vi "DigitalFont.vi"() -> ()   [LabVIEW 2019, in "Digital.lvclass"]
uses:
  Digital.lvclass
  <vilib>/Analysis/coordinate.llb/2D Cartesian Coordinate Rotation (Array).vi
  <vilib>/Analysis/NI_AALPro.lvlib
panel:
  out "Array":T1(array[cluster])
  out "new picture 2":picture
  in  "Numeric":i32
  in  "TopLeft":cluster{"String":dbl, "String":dbl}[](array[cluster])=[{"String"=10.0, "String"=100.0}, {"String"=1.2246467991473533e-15, "String"=80.0}, {"String"=4.898587196589413e-15, "String"=20.0}, {"String"=10.000000000000005, "String"=0.0}, {"String"=20.000000000000004, "String"=20.0}, {"String"=20.0, "String"=80.0}, {"String"=10.0, "String"=100.0}]
  out "appended array":cluster{"String":dbl, "String":dbl}[](array[cluster])
  out "new picture":picture
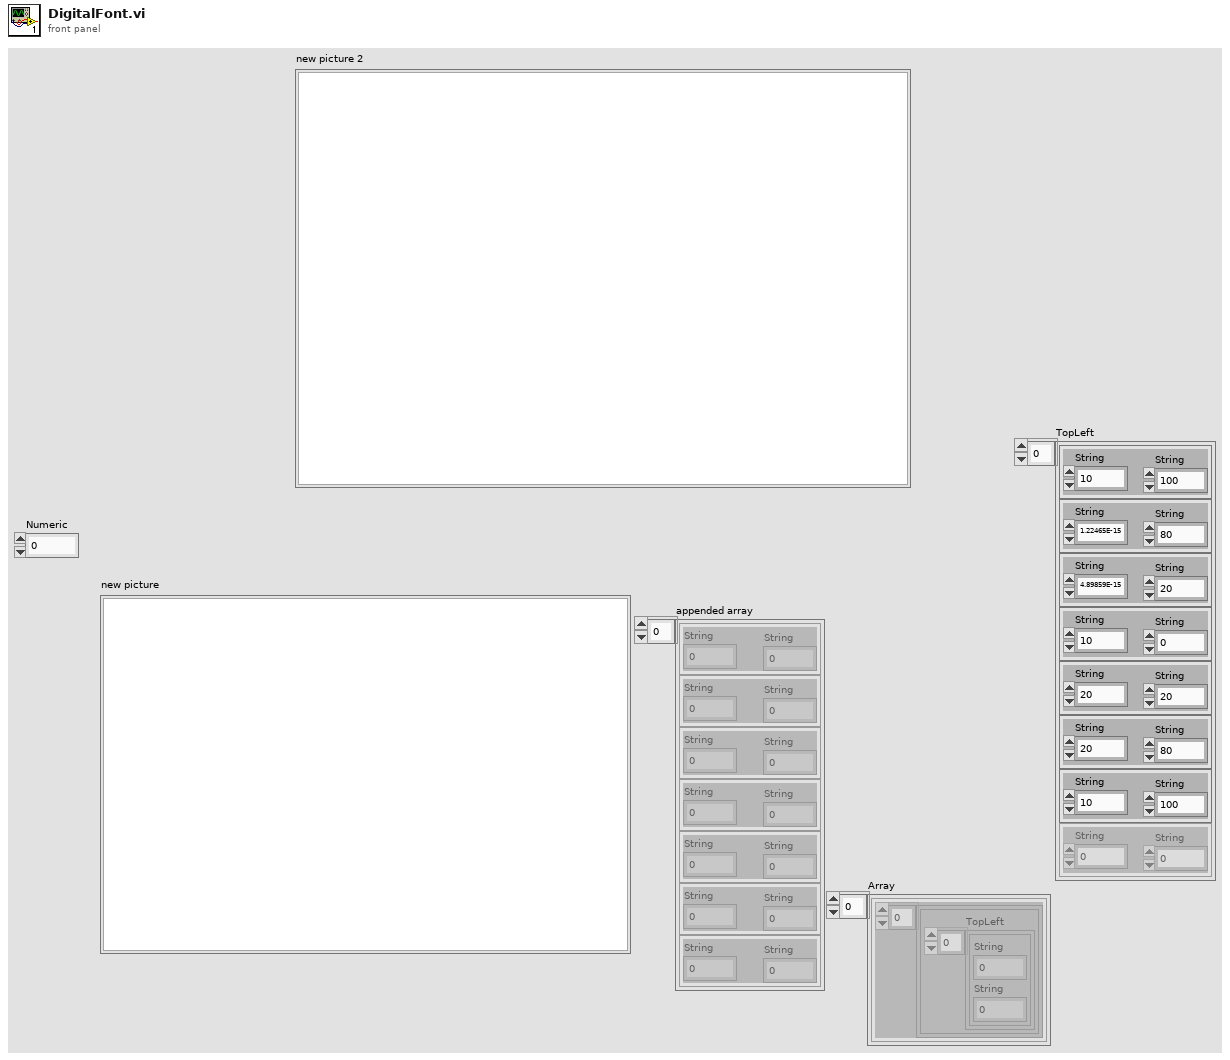
[diagram p1: front panel]
types:
  T1 = cluster{cluster{"TopLeft":cluster{"String":dbl, "String":dbl}[]}[]}[]
  T2 = cluster{"TopLeft":cluster{"String":dbl, "String":dbl}[]}[]
  T3 = cluster{"TopLeft":cluster{"String":dbl, "String":dbl}[]}
  T4 = cluster{"Width":u16, "Style":enum32{"Solid", "Dash", "Dot", "DashDot", "DashDotDot"}}
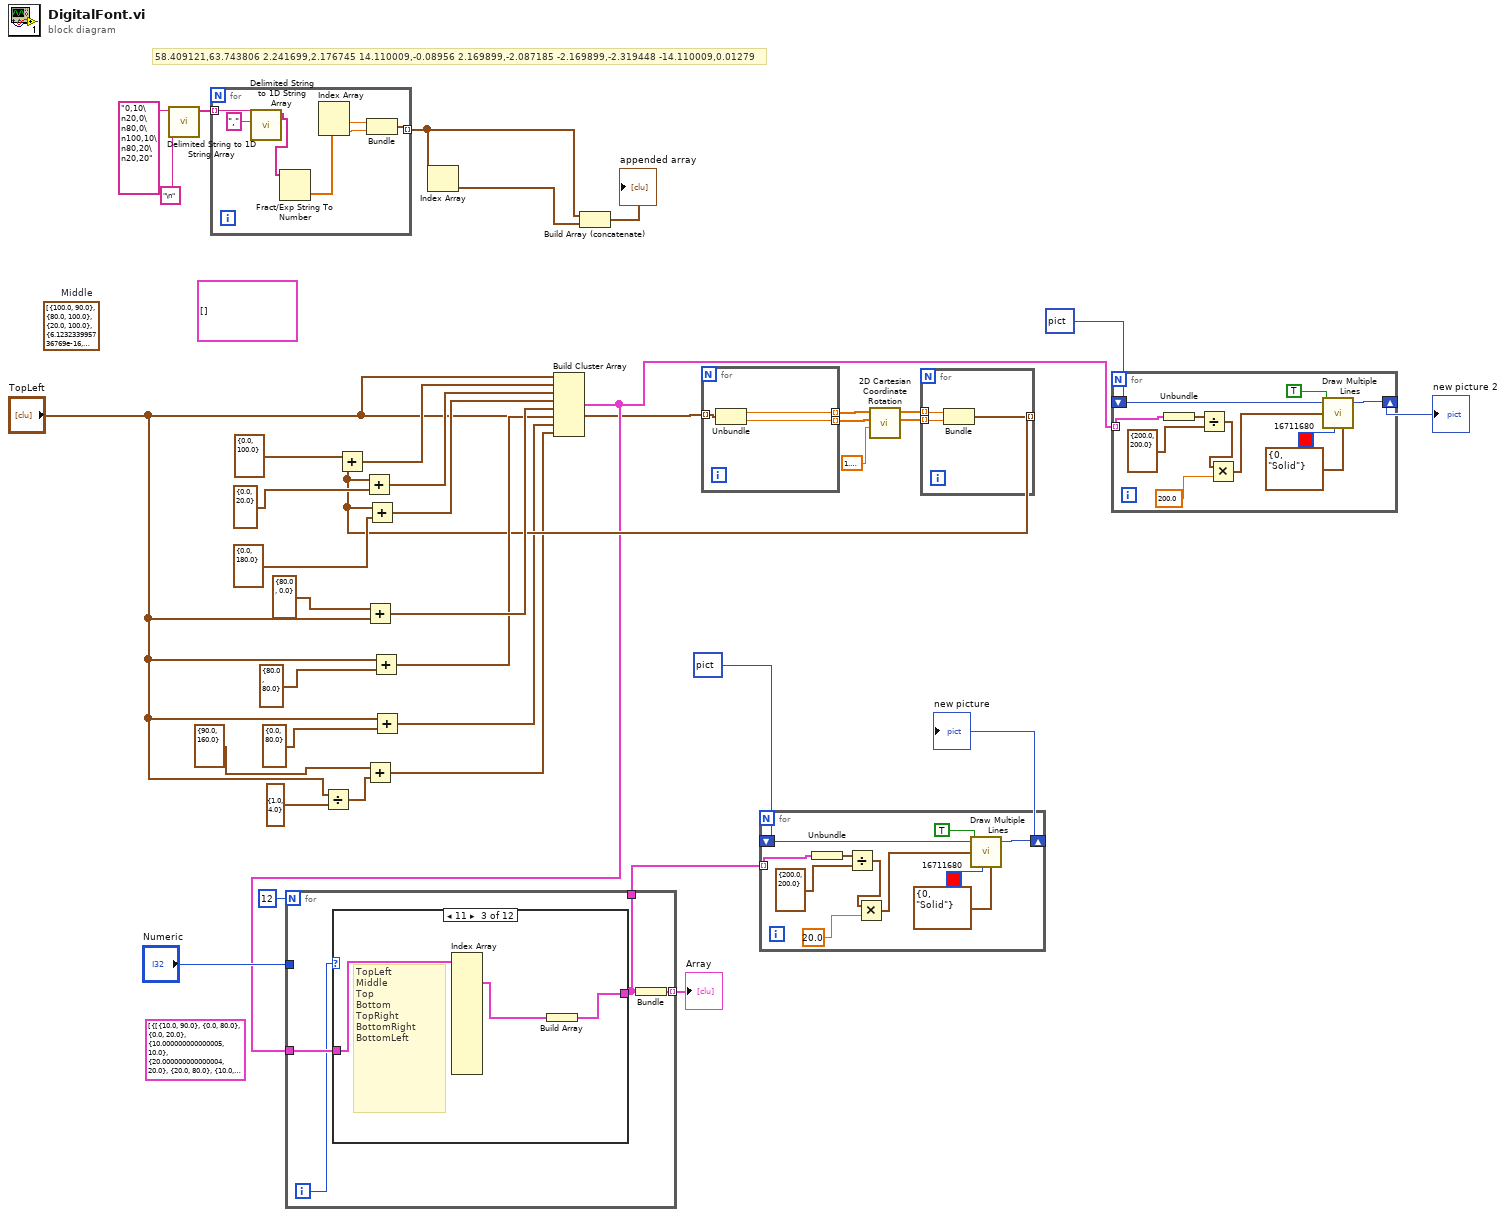
[diagram p0: block diagram]
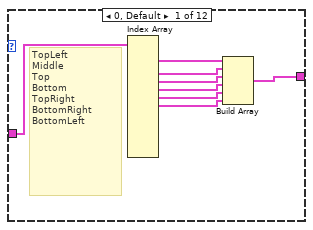
[diagram p2: hidden frame]
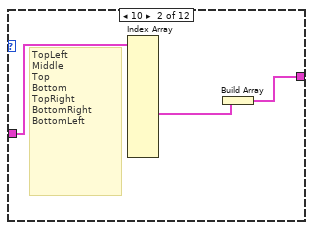
[diagram p3: hidden frame]
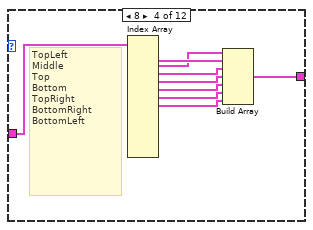
[diagram p4: hidden frame]
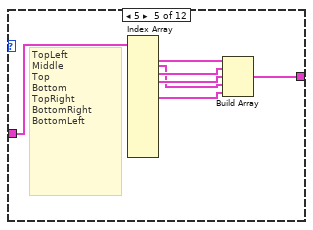
[diagram p5: hidden frame]
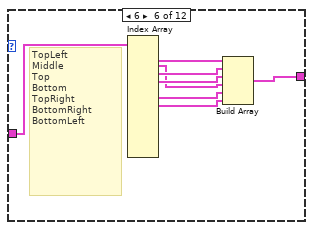
[diagram p6: hidden frame]
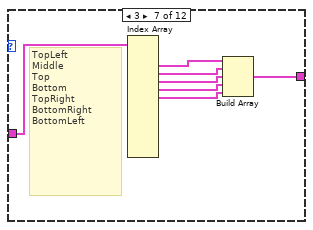
[diagram p7: hidden frame]
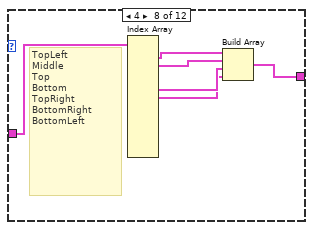
[diagram p8: hidden frame]
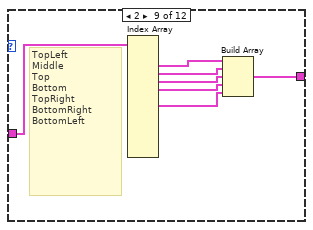
[diagram p9: hidden frame]
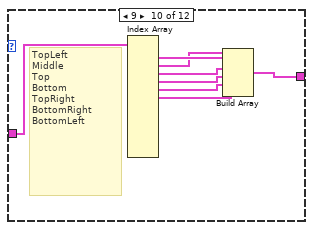
[diagram p10: hidden frame]
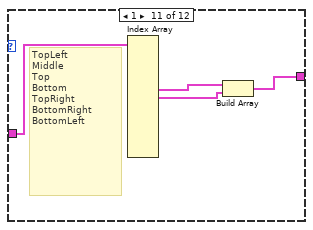
[diagram p11: hidden frame]
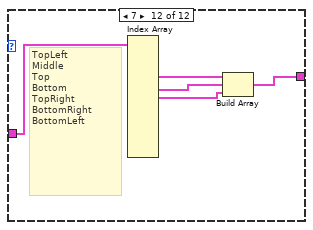
[diagram p12: hidden frame]
diagram:
  (unwired) T2 [{"TopLeft"=[{"String"=10.0, "String"=90.0}, {"String"=0.0, "String"=80.0}, {"String"=0.0, "String"=20.0}, {"String"=10.000000000000005, "String"=10.0}, {"String"=20.000000000000004, "String"=20.0}, {"String"=20.0, "String"=80.0}, {"String"=10.0, "String"=90.0}]}, {"TopLeft"=[{"String"=90.0, "String"=90.0}, {"String"=80.0, "String"=100.0}, {"String"=20.0, "String"=100.0}, {"String"=10.0, "String"=90.0}, {"String"=20.0, "String"=80.0}, {"String"=80.0, "String"=80.0}, {"String"=90.0, "String"=90.0}]}, {"TopLeft"=[{"String"=90.0, "String"=10.000000000000005}, {"String"=80.0, "String"=20.000000000000004}, {"String"=20.0, "String"=20.0}, {"String"=10.0, "String"=9.999999999999995}, {"String"=20.0, "String"=-3.552713678800501e-15}, {"String"=80.0, "String"=3.552713678800501e-15}, {"String"=90.0, "String"=10.000000000000005}]}, {"TopLeft"=[{"String"=90.0, "String"=170.0}, {"String"=80.0, "String"=180.0}, {"String"=20.0, "String"=180.0}, {"String"=10.0, "String"=170.0}, {"String"=20.0, "String"=160.0}, {"String"=80.0, "String"=160.0}, {"String"=90.0, "String"=170.0}]}, {"TopLeft"=[{"String"=90.0, "String"=90.0}, {"String"=80.0, "String"=80.0}, {"String"=80.0, "String"=20.0}, {"String"=90.0, "String"=10.0}, {"String"=100.0, "String"=20.0}, {"String"=100.0, "String"=80.0}, {"String"=90.0, "String"=90.0}]}, {"TopLeft"=[{"String"=90.0, "String"=170.0}, {"String"=80.0, "String"=160.0}, {"String"=80.0, "String"=100.0}, {"String"=90.0, "String"=90.0}, {"String"=100.0, "String"=100.0}, {"String"=100.0, "String"=160.0}, {"String"=90.0, "String"=170.0}]}, {"TopLeft"=[{"String"=10.0, "String"=170.0}, {"String"=0.0, "String"=160.0}, {"String"=0.0, "String"=100.0}, {"String"=10.000000000000005, "String"=90.0}, {"String"=20.000000000000004, "String"=100.0}, {"String"=20.0, "String"=160.0}, {"String"=10.0, "String"=170.0}]}] ("array of clusters")
  (unwired) T2 [] ("array of clusters")
  (unwired) cluster{"String":dbl, "String":dbl}[] [{"String"=100.0, "String"=90.0}, {"String"=80.0, "String"=100.0}, {"String"=20.0, "String"=100.0}, {"String"=6.123233995736769e-16, "String"=90.0}, {"String"=20.0, "String"=80.0}, {"String"=80.0, "String"=80.0}, {"String"=100.0, "String"=90.0}]  # Middle
  # "58.409121,63.743806 2.241699,2.176745 14.110009,-0.08956 2.169899,-2.087185 -2.169899,-2.319448 -14.110009,0.01279"
  n1 = call <vilib>:"Delimited String to 1D String Array.vi"("delimiter"="\n", "delimited string"="0,10\n20,0\n80,0\n100,10\n80,20\n20,20") -> ("string array"=w35:string[])  [unwired: 9 in]
  n2 = for {
    tunnel: w35 -> [w45] mode=indexing
    tunnel: [w39] -> w34 mode=indexing
    n3 = call <vilib>:"Delimited String to 1D String Array.vi"("delimiter"=",", "delimited string"=w45) -> ("string array"=w43:string[])  [unwired: 9 in]
    n4 = Fract/Exp String To Number(string=w43) -> (number=w42:dbl[])  [unwired: 3 in, 1 out]
    n5 = Index Array(array=w42) -> (element #1=w41:dbl, element #2=w40:dbl)  [unwired: 2 in]
    n6 = Bundle("String"=w41, "String"=w40) -> (w39:cluster{"String":dbl, "String":dbl})  [unwired: 1 in]
  }
  n7 = Divide(x="TopLeft", y=cluster{"String":dbl, "String":dbl} {"String"=1.0, "String"=4.0} ("output cluster")) -> (x/y=w5:cluster{"String":dbl, "String":dbl}[])
  n8 = Add(x=cluster{"String":dbl, "String":dbl} {"String"=80.0, "String"=0.0} ("output cluster"), y="TopLeft") -> (x+y=w18:cluster{"String":dbl, "String":dbl}[])
  n9 = Add(x=cluster{"String":dbl, "String":dbl} {"String"=90.0, "String"=160.0} ("output cluster"), y=w5) -> (x+y=w3:cluster{"String":dbl, "String":dbl}[])
  n10 = Add(x="TopLeft", y=cluster{"String":dbl, "String":dbl} {"String"=80.0, "String"=80.0} ("output cluster")) -> (x+y=w16:cluster{"String":dbl, "String":dbl}[])
  n11 = Add(x="TopLeft", y=cluster{"String":dbl, "String":dbl} {"String"=0.0, "String"=80.0} ("output cluster")) -> (x+y=w8:cluster{"String":dbl, "String":dbl}[])
  n12 = Index Array(array=w34) -> (element=w33:cluster{"String":dbl, "String":dbl})  [unwired: 1 in]
  n13 = Build Array (concatenate)(w34, w33) -> (→"appended array":cluster{"String":dbl, "String":dbl}[])
  n14 = for {
    tunnel: "TopLeft" -> [w48] mode=indexing
    tunnel: [w47] -> w32 mode=indexing
    tunnel: [w46] -> w31 mode=indexing
    n15 = Unbundle(w48) -> ("String"=w47:dbl, "String"=w46:dbl)
  }
  n16 = call-poly <vilib>:"2D Cartesian Coordinate Rotation.vi"("theta"=1.5707963267948966, "Y"=w31, "X"=w32) -> ("Y Out"=w29:dbl[], "X Out"=w30:dbl[])  [unwired: 6 in, 1 out]
  n17 = for {
    tunnel: w30 -> [w50] mode=indexing
    tunnel: w29 -> [w51] mode=indexing
    tunnel: [w49] -> w10 mode=indexing
    n18 = Bundle("Numeric"=w50, "Numeric"=w51) -> (w49:cluster{"Numeric":dbl, "Numeric":dbl})  [unwired: 1 in]
  }
  n19 = Add(x=cluster{"String":dbl, "String":dbl} {"String"=0.0, "String"=100.0} ("output cluster"), y=w10) -> (x+y=w25:cluster{dbl, dbl}[])
  n20 = Add(x=w10, y=cluster{"String":dbl, "String":dbl} {"String"=0.0, "String"=20.0} ("output cluster")) -> (x+y=w22:cluster{dbl, dbl}[])
  n21 = Add(x=w10, y=cluster{"String":dbl, "String":dbl} {"String"=0.0, "String"=180.0} ("output cluster")) -> (x+y=w20:cluster{dbl, dbl}[])
  n22 = Build Cluster Array("TopLeft", w25, w22, w20, w18, w16, w8, w3) -> (w9:T2)
  n23 = for {
    N: 12 -> [_]
    tunnel: w9 -> [w55]
    tunnel: "Numeric" -> [_]
    tunnel: [w53] -> w13
    tunnel: [w52] -> w1 mode=indexing
    i -> [w54]
    n24 = case shown="11" w54 {
      tunnel: w55 -> [w63 w66 w69 w78 w85 w93 w100 w106 w113 w121 w125 w130]
      tunnel: [w57 w65 w68 w72 w81 w89 w95 w103 w110 w118 w123 w128] -> w53
      frame 0, Default {
        # "TopLeft\nMiddle\nTop\nBottom\nTopRight\nBottomRight\nBottomLeft"
        n25 = Index Array(array=w63) -> (element #1=w62:T3, element #3=w61:T3, element #4=w60:T3, element #5=w59:T3, element #6=w58:T3, element #7=w56:T3)  [unwired: 13 in, 7 out]
        n26 = Build Array(w62, w61, w60, w59, w58, w56) -> (w57:T2)
      }
      frame 10 {
        # "TopLeft\nMiddle\nTop\nBottom\nTopRight\nBottomRight\nBottomLeft"
        n27 = Index Array(array=w66) -> (element #8=w64:T3)  [unwired: 13 in, 12 out]
        n28 = Build Array(w64) -> (w65:T2)
      }
      frame 11 {
        # "TopLeft\nMiddle\nTop\nBottom\nTopRight\nBottomRight\nBottomLeft"
        n29 = Index Array(array=w69) -> (element #2=w67:T3)  [unwired: 13 in, 12 out]
        n30 = Build Array(w67) -> (w68:T2)
      }
      frame 8 {
        # "TopLeft\nMiddle\nTop\nBottom\nTopRight\nBottomRight\nBottomLeft"
        n31 = Index Array(array=w78) -> (element #1=w77:T3, element #2=w70:T3, element #3=w76:T3, element #4=w75:T3, element #5=w74:T3, element #6=w73:T3, element #7=w71:T3)  [unwired: 13 in, 6 out]
        n32 = Build Array(w70, w77, w76, w75, w74, w73, w71) -> (w72:T2)
      }
      frame 5 {
        # "TopLeft\nMiddle\nTop\nBottom\nTopRight\nBottomRight\nBottomLeft"
        n33 = Index Array(array=w85) -> (element #1=w84:T3, element #2=w79:T3, element #3=w83:T3, element #4=w82:T3, element #6=w80:T3)  [unwired: 13 in, 8 out]
        n34 = Build Array(w84, w83, w82, w79, w80) -> (w81:T2)
      }
      frame 6 {
        # "TopLeft\nMiddle\nTop\nBottom\nTopRight\nBottomRight\nBottomLeft"
        n35 = Index Array(array=w93) -> (element #1=w92:T3, element #2=w87:T3, element #3=w91:T3, element #4=w90:T3, element #6=w88:T3, element #7=w86:T3)  [unwired: 13 in, 7 out]
        n36 = Build Array(w92, w91, w90, w87, w88, w86) -> (w89:T2)
      }
      frame 3 {
        # "TopLeft\nMiddle\nTop\nBottom\nTopRight\nBottomRight\nBottomLeft"
        n37 = Index Array(array=w100) -> (element #2=w94:T3, element #3=w99:T3, element #4=w98:T3, element #5=w97:T3, element #6=w96:T3)  [unwired: 13 in, 8 out]
        n38 = Build Array(w94, w99, w98, w97, w96) -> (w95:T2)
      }
      frame 4 {
        # "TopLeft\nMiddle\nTop\nBottom\nTopRight\nBottomRight\nBottomLeft"
        n39 = Index Array(array=w106) -> (element #1=w101:T3, element #2=w102:T3, element #5=w105:T3, element #6=w104:T3)  [unwired: 13 in, 9 out]
        n40 = Build Array(w101, w102, w105, w104) -> (w103:T2)
      }
      frame 2 {
        # "TopLeft\nMiddle\nTop\nBottom\nTopRight\nBottomRight\nBottomLeft"
        n41 = Index Array(array=w113) -> (element #2=w109:T3, element #3=w112:T3, element #4=w111:T3, element #5=w108:T3, element #7=w107:T3)  [unwired: 13 in, 8 out]
        n42 = Build Array(w109, w112, w111, w108, w107) -> (w110:T2)
      }
      frame 9 {
        # "TopLeft\nMiddle\nTop\nBottom\nTopRight\nBottomRight\nBottomLeft"
        n43 = Index Array(array=w121) -> (element #1=w115:T3, element #2=w114:T3, element #3=w120:T3, element #4=w119:T3, element #5=w117:T3, element #6=w116:T3)  [unwired: 13 in, 7 out]
        n44 = Build Array(w114, w115, w120, w119, w117, w116) -> (w118:T2)
      }
      frame 1 {
        # "TopLeft\nMiddle\nTop\nBottom\nTopRight\nBottomRight\nBottomLeft"
        n45 = Index Array(array=w125) -> (element #5=w122:T3, element #6=w124:T3)  [unwired: 13 in, 11 out]
        n46 = Build Array(w122, w124) -> (w123:T2)
      }
      frame 7 {
        # "TopLeft\nMiddle\nTop\nBottom\nTopRight\nBottomRight\nBottomLeft"
        n47 = Index Array(array=w130) -> (element #3=w126:T3, element #5=w127:T3, element #6=w129:T3)  [unwired: 13 in, 10 out]
        n48 = Build Array(w126, w127, w129) -> (w128:T2)
      }
    }
    n49 = Bundle(w53) -> (w52:cluster{cluster{"TopLeft":cluster[]}[]})  [unwired: 1 in]
  }
  "Array" <- w1
  n50 = for {
    shift-right: [w141] -> w38
    shift-left: picture data[5B] ("new picture") -> [w137]
    tunnel: w13 -> [w136] mode=indexing
    n51 = Unbundle(w136) -> ("TopLeft"=w134:cluster{"String":dbl, "String":dbl}[])
    n52 = Divide(x=w134, y=cluster{"String":dbl, "String":dbl} {"String"=200.0, "String"=200.0}) -> (x/y=w132:cluster{"String":dbl, "String":dbl}[])
    n53 = Multiply(x=w132, y=20.0 ("String")) -> (x*y=w131:cluster{"String":dbl, "String":dbl}[])
    n54 = call <vilib>:"Draw Multiple Lines.vi"("picture"=w137, "line endpoints"=w131, "fill?(F)"=TRUE, "color(black)"=u32 16711680, "pen"=T4 {"Width"=0, "Style"=enum."Solid"}) -> ("new picture"=w141:picture)  [unwired: 4 in]
  }
  "new picture" <- w38
  n55 = for {
    shift-right: [w152] -> w11
    shift-left: picture data[5B] ("new picture") -> [w148]
    tunnel: w9 -> [w147] mode=indexing
    n56 = Unbundle(w147) -> ("TopLeft"=w145:cluster{"String":dbl, "String":dbl}[])
    n57 = Divide(x=w145, y=cluster{"String":dbl, "String":dbl} {"String"=200.0, "String"=200.0}) -> (x/y=w143:cluster{"String":dbl, "String":dbl}[])
    n58 = Multiply(x=w143, y=200.0 ("String")) -> (x*y=w142:cluster{"String":dbl, "String":dbl}[])
    n59 = call <vilib>:"Draw Multiple Lines.vi"("picture"=w148, "line endpoints"=w142, "fill?(F)"=TRUE, "color(black)"=u32 16711680, "pen"=T4 {"Width"=0, "Style"=enum."Solid"}) -> ("new picture"=w152:picture)  [unwired: 4 in]
  }
  "new picture 2" <- w11
